vi "savingPrepDataForDisp.vi"(7 "save":bool, 8 "error in (no error)":errorcluster, 9 "buffer in":i16[](array[numeric]), 10 "Channels to read":i32, 11 "Byte Stream File in":refnum<file>) -> (0 "error out":errorcluster, 2 "Array":dbl[][](array[numeric]), 3 "Byte Stream File out":refnum<file>, 4 "function return":u32(ring))   [LabVIEW 2021]
uses:
  <userlib>/er4commlib_labview/er4commlib_labview.lvlib
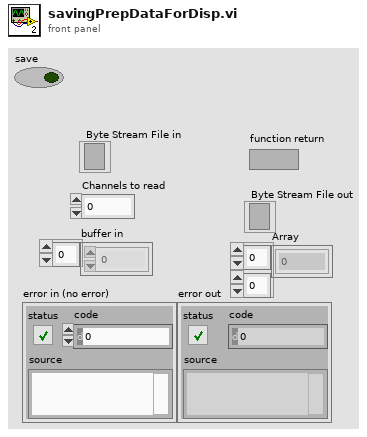
[diagram p1: front panel]
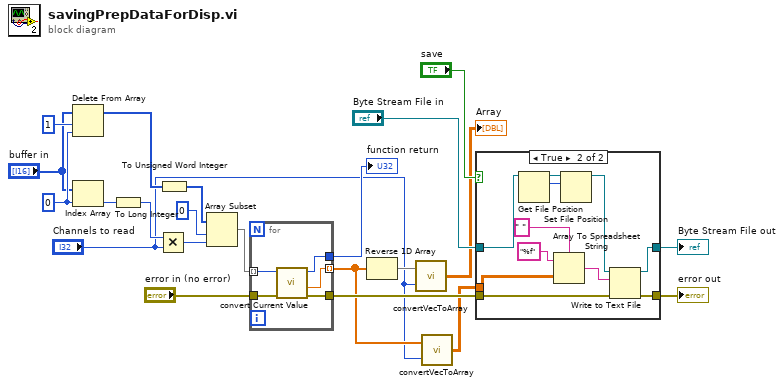
[diagram p0: block diagram]
diagram:
  w17 = 0 ("index")
  n1 = Delete From Array(array="buffer in", length=1, index=w17) -> (array with subset deleted=w18:i16[])  [unwired: 1 out]
  n2 = Index Array(array="buffer in", index=w17) -> (element=w6:i16)
  n3 = To Long Integer(number=w6) -> (32bit integer=w7:i32)
  n4 = Multiply(x=w7, y="Channels to read") -> (x*y=w8:i32)
  n5 = To Unsigned Word Integer(number=w18) -> (unsigned 16bit integer=w9:u16[])
  n6 = Array Subset(array=w9, index=0, length=w8) -> (w5:u16[])
  n7 = for {
    tunnel: w5 -> [w27] mode=indexing
    tunnel: [w24] -> w3 mode=indexing
    tunnel: "error in (no error)" -> [w26]
    tunnel: [w25] -> w21
    tunnel: [w23] -> w10
    n8 = call <userlib>:"convert Current Value.vi"("error in (no error)"=w26, "intValue"=w27) -> ("error out"=w25:errorcluster, "fltValue out"=w24:dbl, "function return"=w23:u32)  [unwired: 7 in]
  }
  "function return" <- w10
  n9 = Reverse 1D Array(array=w3) -> (reversed array=w4:dbl[])
  n10 = call "convertVecToArray.vi"("Channels"="Channels to read", "buffer in"=w4) -> ("Array"=→"Array":dbl[][])
  n11 = call "convertVecToArray.vi"("Channels"="Channels to read", "buffer in"=w3) -> ("Array"=w1:dbl[][])
  n12 = case shown="True" "save" {
    tunnel: [w28 w40] -> w22
    tunnel: w21 -> [w28 w39]
    tunnel: "Byte Stream File in" -> [w29 w38]
    tunnel: [w29 w32] -> w15
    tunnel: w1 -> [_ w30]
    frame False {
    }
    frame True {
      n13 = Get File Position(7:w38) -> (2:w37:i64, 3:w36:refnum<file>)  [unwired: 1 in, 1 out]
      n14 = Array To Spreadsheet String(delimiter (Tab)=" ", array=w30, 3:"%f" ("format string")) -> (spreadsheet string=w31:string)
      n15 = Set File Position(offset (in bytes) (0)=w37, refnum=w36) -> (refnum out=w35:refnum<file>)  [unwired: 2 in, 1 out]
      n16 = Write to Text File(file (use dialog)=w35, text=w31, error in=w39) -> (refnum out=w32:refnum<file>, error out=w40:errorcluster)  [unwired: 1 in, 1 out]
    }
  }
  "error out" <- w22
  "Byte Stream File out" <- w15
